vi "AutoTurn.vi"(9 "Steady Val":dbl, 11 "Degrees to turn":dbl) -> ()   [LabVIEW 2012]
uses:
  StateMachineEnum.ctl
  Robot Global Data.vi
  <vilib>/Rock Robotics/WPI/RobotDrive/WPI_RobotDriveGetSetRefNum.vi
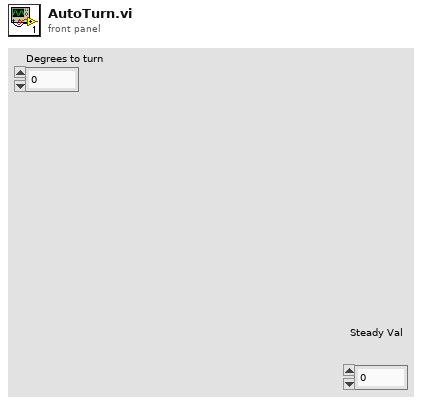
[diagram p1: front panel]
types:
  T1 = typedef "StateMachineEnum.ctl" = enum16{"Init", "Idle", "Start", "Do", "Stop"}
  T2 = typedef "WPI_GyroDevRef.ctl" = cluster{"DevStatus":errorcluster, "Analog Module":T3, "Analog Channel":T4, "Offset":dbl, "Gain (VoltsPerDegree/Second)":dbl}
  T3 = typedef "FPGA_TypedefAnalogModule.ctl" = enum16{"Analog Module 1", "Analog Module 2"}
  T4 = typedef "FPGA_AIChannel.ctl" = enum8{"AI 1", "AI 2", "AI 3", "AI 4", "AI 5", "AI 6", "AI 7", "AI 8", "Invalid"}
  T5 = typedef "WPI_RobotDriveDevRef.ctl" = cluster{"DevStatus":errorcluster, "Motors[]":T6[], "Square Inputs":bool, "Max Output":dbl, "Isochronous":bool}
  T6 = typedef "WPI_MotorControlDeviceRef.ctl" = cluster{"DeviceStatus":errorcluster, "Type":enum16{"PWM", "CAN"}, "PWM":cluster{"Digital Module":T7, "PWM Channel":T8, "DeadBand":T9}, "CAN":cluster{"Device Number":u8, "Control Mode":T10, "Semaphore":T11, "Max Vout":dbl}, "Invert":bool, "TransformRef":T12, "InvTransformRef":T12}
  T7 = typedef "FPGA_TypedefDigitalModule.ctl" = enum16{"Digital Module 1", "Digital Module 2"}
  T8 = typedef "FPGA_DIOPWMChannel.ctl" = enum8{"PWM 1", "PWM 2", "PWM 3", "PWM 4", "PWM 5", "PWM 6", "PWM 7", "PWM 8", "PWM 9", "PWM 10", "Invalid"}
  T9 = typedef "WPI_PWMDeadband.ctl" = cluster{"Name":string, "maxPositivePwm":i32, "minPositivePwm":i32, "centerPwm":i32, "maxNegativePwm":i32, "minNegativePwm":i32, "angularRange":u16}
  T10 = typedef "WPI_CANJaguar_ControlMode.ctl" = enum8{"Percent VBus", "Current", "Speed", "Position", "Voltage"}
  T11 = typedef "Semaphore RefNum" = refnum<k1>
  T12 = typedef "WPI_PWMTransform_ConPane.ctl" = refnum<vi>
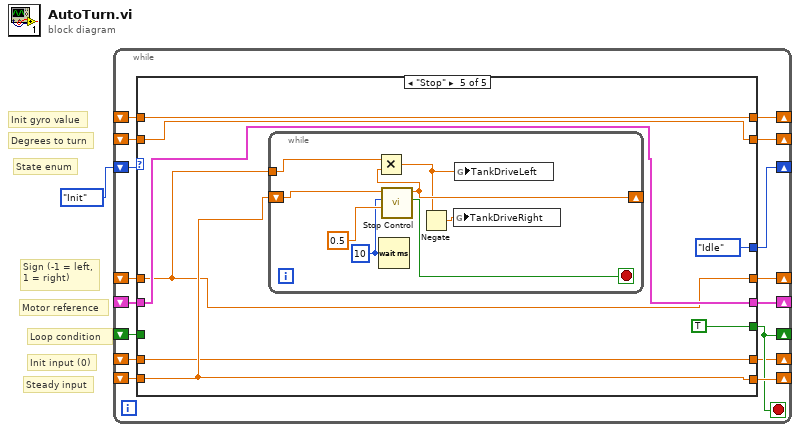
[diagram p0: block diagram]
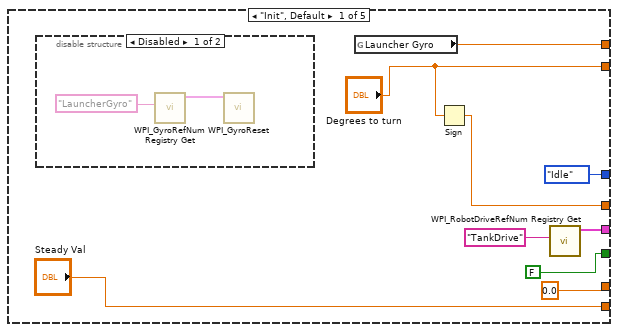
[diagram p2: hidden frame]
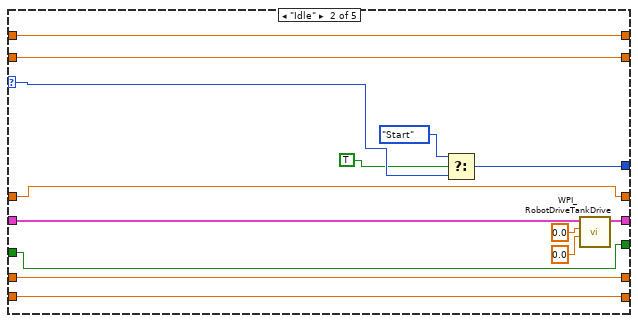
[diagram p4: hidden frame]
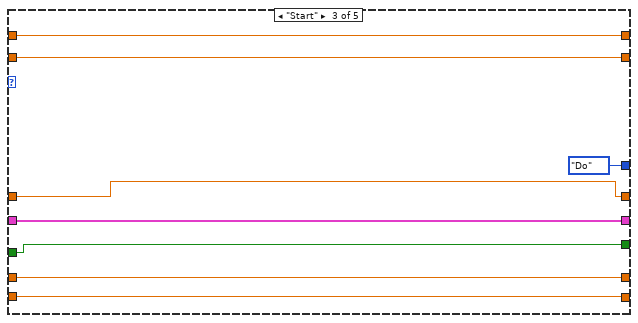
[diagram p5: hidden frame]
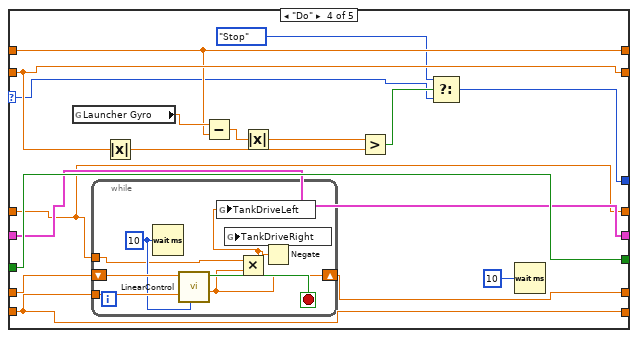
[diagram p6: hidden frame]
diagram:
  # "Sign (-1 = left,\n1 = right)"
  # "Degrees to turn"
  # "Init gyro value"
  # "State enum"
  # "Motor reference"
  # "Loop condition"
  # "Init input (0)"
  # "Steady input"
  n1 = while {
    shift-right: [w14] -> _
    shift-left: StateMachineEnum."Init" -> [w17]
    shift-right: [w16] -> _
    shift-left: _ -> [w15]
    shift-right: [w13] -> _
    shift-left: _ -> [w12]
    shift-right: [w11] -> _
    shift-left: _ -> [w10]
    shift-right: [w9] -> _
    shift-left: _ -> [w7]
    shift-right: [w8] -> _
    shift-left: _ -> [w6]
    shift-right: [w5] -> _
    shift-left: _ -> [w4]
    shift-right: [w3] -> _
    shift-left: _ -> [w2]
    stop <- w11 stop-if-true
    n2 = case shown="\"Stop\"" w17 {
      selector: w17 -> [_ w36 _ w53 _]
      tunnel: [w25 w37 w49 w63 w80] -> w16
      tunnel: w15 -> [_ w39 w49 w63 w80]
      tunnel: [StateMachineEnum."Idle" w42 StateMachineEnum."Do" w67 StateMachineEnum."Idle" ("f")] -> w14
      tunnel: ["Steady Val" w34 w48 w65 w82] -> w13
      tunnel: w12 -> [_ w34 w48 w65 w82]
      tunnel: [FALSE w33 w47 w64 TRUE] -> w11
      tunnel: w10 -> [_ w33 w47 w64 _]
      tunnel: [0.0 ("Right axis value") w32 w45 w60 w79] -> w9
      tunnel: [w20 w31 w46 w54 w78] -> w8
      tunnel: w7 -> [_ w32 w45 w61 w79]
      tunnel: w6 -> [_ w31 w46 w54 w78]
      tunnel: ["Degrees to turn" w30 w44 w55 w77] -> w5
      tunnel: w4 -> [_ w30 w44 w55 w77]
      tunnel: [w18 w29 w43 w51 w76] -> w3
      tunnel: w2 -> [_ w29 w43 w51 w76]
      frame "Init", Default {
        n3 = disable-structure shown="Disabled" {
          frame Disabled {
            n4 = call <vilib>:"WPI_GyroRefNum Registry Get.vi"("refnum name"="LauncherGyro") -> ("GyroDevRef"=w27:T2)  [unwired: 9 in, 1 out]
            n5 = call <vilib>:"WPI_GyroReset.vi"("GyroDevRef"=w27) -> ()  [unwired: 9 in, 2 out]
          }
          frame Enabled {
          }
        }
        n6 = global read "Robot Global Data.vi" "Launcher Gyro"() -> (w20:dbl)
        n7 = Sign(1:"Degrees to turn") -> (0:w18:dbl)
        n8 = call <vilib>:"WPI_RobotDriveRefNum Registry Get.vi"("refnum name"="TankDrive") -> ("RobotDriveDevRef"=w25:T5)  [unwired: 9 in, 1 out]
      }
      frame "Idle" {
        n9 = Select(t=StateMachineEnum."Start", s=TRUE, f=w36) -> (s? t:f=w42:T1)
        n10 = call <vilib>:"WPI_RobotDriveTankDrive.vi"("Right axis value"=0.0, "Left axis value"=0.0, "RobotDriveDevRef"=w39) -> ("RobotDriveDevRef"=w37:T5)  [unwired: 6 in, 2 out]
      }
      frame "Start" {
      }
      frame "Do" {
        n11 = global read "Robot Global Data.vi" "Launcher Gyro"() -> (w58:dbl)
        n12 = while {
          shift-right: [w71] -> w60
          shift-left: w61 -> [w74]
          tunnel: w65 -> [w73]
          tunnel: w51 -> [w70]
          stop <- w75 stop-if-true
          w72 = u32 10 ("milliseconds to wait")
          n13 = Wait (ms)(milliseconds to wait=w72) -> ()  [unwired: 1 out]
          n14 = call "LinearControl.vi"("Loop Time (ms)"=w72, "Setpoint"=w73, "Recieved Motor Input"=w74) -> ("New Motor Input"=w71:dbl, "Currently Matching"=w75:bool)  [unwired: 7 in]
          n15 = Multiply(x=w70, y=w71) -> (x*y=w68:dbl)
          n16 = global write "Robot Global Data.vi" "TankDriveLeft"(w68) -> ()
          n17 = Negate(x=w68) -> (-x=w69:dbl)
          n18 = global write "Robot Global Data.vi" "TankDriveRight"(w69) -> ()
        }
        n19 = Absolute Value(x=w55) -> (abs(x)=w56:dbl)
        n20 = Subtract(x=w58, y=w54) -> (x-y=w59:dbl)
        n21 = Absolute Value(x=w59) -> (abs(x)=w57:dbl)
        n22 = Greater?(x=w57, y=w56) -> (0:w62:bool)
        n23 = Select(t=StateMachineEnum."Stop" ("f"), s=w62, f=w53) -> (s? t:f=w67:T1)
        n24 = Wait (ms)(milliseconds to wait=u32 10) -> ()  [unwired: 1 out]
      }
      frame "Stop" {
        n25 = while {
          shift-right: [w86] -> _
          shift-left: w82 -> [w90]
          tunnel: w76 -> [w87]
          stop <- w89 stop-if-true
          w88 = u32 10 ("milliseconds to wait")
          n26 = Wait (ms)(milliseconds to wait=w88) -> ()  [unwired: 1 out]
          n27 = call "Stop Control.vi"("Rate (unit/s)"=0.5, "Loop Time (ms)"=w88, "Recieved Motor Input"=w90) -> ("Done Stopping"=w89:bool, "New Motor Input"=w86:dbl)  [unwired: 7 in]
          n28 = Multiply(x=w87, y=w86) -> (x*y=w85:dbl)
          n29 = Negate(x=w85) -> (-x=w84:dbl)
          n30 = global write "Robot Global Data.vi" "TankDriveRight"(w84) -> ()
          n31 = global write "Robot Global Data.vi" "TankDriveLeft"(w85) -> ()
        }
      }
    }
  }
